vi "Config.vi"(8 "error in (no error)":errorcluster, 10 "Setting":variant, 11 "NI Digitizer in":refnum<class "NI Digitizer.lvclass">) -> (0 "error out":errorcluster, 3 "NI Digitizer out":refnum<class "NI Digitizer.lvclass">)   [LabVIEW 2025, in "Digitizer.lvlib" / "NI Digitizer.lvclass"]
uses:
  NI Digitizer.lvclass
  Digitizer configuration/Digitizer configuration.lvclass
  NI Digitizer.lvclass/NI Digitizer.ctl
  Digitizer configuration/Digitizer configuration.lvclass/Digitizer configuration.ctl
  Users/Public/Documents/Sandia National Labs/TSS Plugin/CEF.lvlibp/serializable configuration/CEF_serializable configuration.lvclass
  <vilib>/DAQmx/configure/trigger.llb/DAQmx Start Trigger (None).vi
  <vilib>/DAQmx/configure/trigger.llb/DAQmx Reference Trigger (None).vi
  <vilib>/DAQmx/configure/timing.llb/DAQmx Timing (Sample Clock).vi
  <resource>/objmgr/daqmx.rc
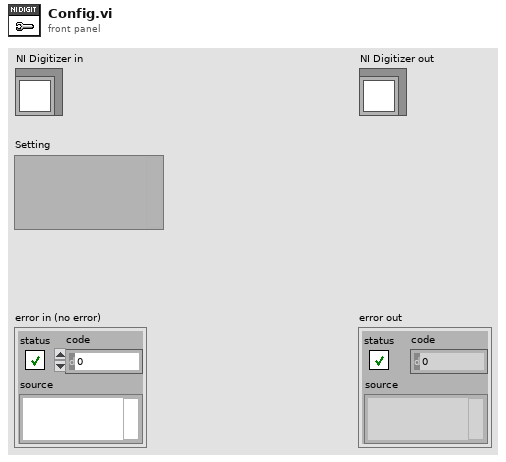
[diagram p1: front panel]
types:
  T1 = typedef "Digitizer.lvlib/Digitizer configuration.lvclass/Digitizer Instrument Setting.ctl" = cluster{"SampleMode":string, "SampleDuration":dbl, "SampleRate":u32, "ReferenceClock":string, "SampleClockEdge":string, "TrigType":string, "TrigLevel":dbl, "TrigSource":string, "Pretrigger":dbl, "TrigDest":string}
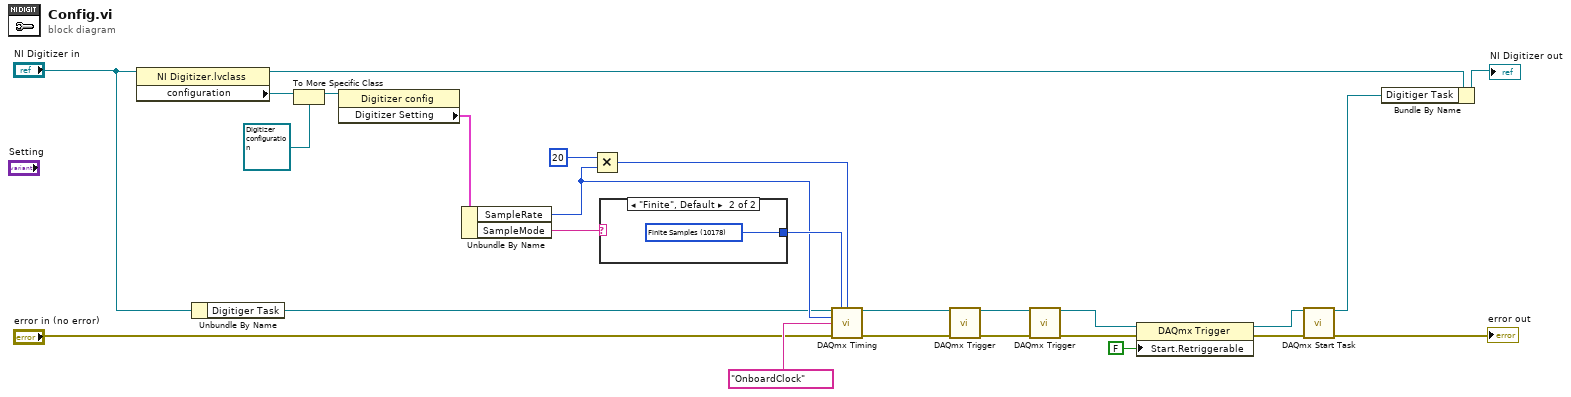
[diagram p0: block diagram]
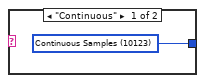
[diagram p2: hidden frame]
diagram:
  n1 = property class="NI Digitizer.lvclass"(reference="NI Digitizer in") -> (reference out=w7:refnum<class "NI Digitizer.lvclass">, "configuration"=w6:refnum<class "CEF_serializable configuration.lvclass">)  [unwired: 1 in, 1 out]
  n2 = Unbundle By Name("NI Digitizer in") -> ("Digitiger Task"=w3:refnum<k21>)
  n3 = To More Specific Class(target class=refnum<class "Digitizer configuration.lvclass"> refnum ("Digitizer.lvlib:Digitizer configuration.lvclass"), reference=w6) -> (specific class reference=w4:refnum<class "Digitizer configuration.lvclass">)  [unwired: 1 in, 1 out]
  n4 = property class="Digitizer config"(reference=w4) -> ("Digitizer Setting"=w1:T1)  [unwired: 1 in, 2 out]
  n5 = Unbundle By Name(w1) -> ("SampleRate"=w24:u32, "SampleMode"=w25:string)
  n6 = Multiply(x=20 ("value"), y=w24) -> (x*y=w23:u32)
  n7 = case shown="\"Finite\", Default" w25 {
    tunnel: [w27 w28] -> w26
    frame "Continuous" {
      w27 = 10123 items=["Finite Samples"=10178, "Continuous Samples"=10123, "Hardware Timed Single Point"=12522] ("sample mode")
    }
    frame "Finite", Default {
      w28 = 10178 items=["Finite Samples"=10178, "Continuous Samples"=10123, "Hardware Timed Single Point"=12522] ("sample mode")
    }
  }
  n8 = call-poly <vilib>:"DAQmx Timing.vi"("task/channels in"=w3, "sample mode"=w26, "samples per channel"=w23, "rate"=w24, "source"=tag "OnboardClock", "error in"="error in (no error)") -> ("task out"=w20:refnum<k21>, "error out"=w18:errorcluster)  [unwired: 8 in]
  n9 = call-poly <vilib>:"DAQmx Trigger.vi"("task/channels in"=w20, "error in"=w18) -> ("task out"=w17:refnum<k21>, "error out"=w16:errorcluster)  [unwired: 12 in]
  n10 = call-poly <vilib>:"DAQmx Trigger.vi"("task/channels in"=w17, "error in"=w16) -> ("task out"=w14:refnum<k21>, "error out"=w13:errorcluster)  [unwired: 12 in]
  n11 = property class="DAQmx Trigger"(reference=w14, error in=w13, "Start.Retriggerable"=FALSE) -> (reference out=w21:refnum<k21>, error out=w19:errorcluster)
  n12 = call <vilib>:"DAQmx Start Task.vi"("task/channels in"=w21, "error in"=w19) -> ("task out"=w9:refnum<k21>, "error out"=→"error out":errorcluster)  [unwired: 12 in]
  n13 = Bundle By Name(cluster=w7, "Digitiger Task"=w9) -> (→"NI Digitizer out":refnum<class "NI Digitizer.lvclass">)
